vi "TestStand_Control ( Close_Seq ).vi"(8 "error in (no error)":errorcluster, 11 "TestStand UI Data":T1) -> (0 "error out":errorcluster)   [LabVIEW 2018, in "TestStand_Control.lvlib"]
uses:
  Module_Controls/TestStand UI Data.ctl
  TestStand_Control.lvlib
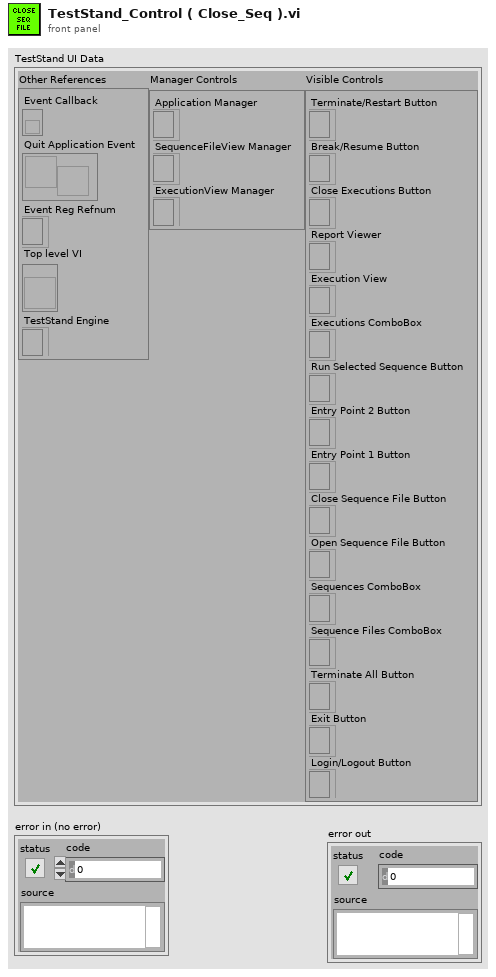
[diagram p1: front panel]
types:
  T1 = typedef "TestStand_Control.lvlib/TestStand UI Data.ctl" = cluster{"Other References":cluster{"Event Callback":refnum<k27>, "Quit Application Event":refnum<user-event>, "Event Reg Refnum":refnum<event-registration>, "Top level VI":refnum<vi>, "TestStand Engine":refnum<k7>}, "Manager Controls":cluster{"Application Manager":refnum<k7>, "SequenceFileView Manager":refnum<k7>, "ExecutionView Manager":refnum<k7>}, "Visible Controls":cluster{"Terminate/Restart Button":refnum<k7>, "Break/Resume Button":refnum<k7>, "Close Executions Button":refnum<k7>, "Report Viewer":refnum<k7>, "Execution View":refnum<k7>, "Executions ComboBox":refnum<k7>, "Run Selected Sequence Button":refnum<k7>, "Entry Point 2 Button":refnum<k7>, "Entry Point 1 Button":refnum<k7>, "Close Sequence File Button":refnum<k7>, "Open Sequence File Button":refnum<k7>, "Sequences ComboBox":refnum<k7>, "Sequence Files ComboBox":refnum<k7>, "Terminate All Button":refnum<k7>, "Exit Button":refnum<k7>, "Login/Logout Button":refnum<k7>}}
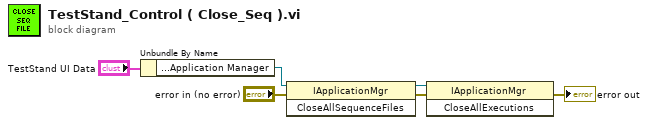
[diagram p0: block diagram]
diagram:
  n1 = Unbundle By Name("TestStand UI Data") -> ("Manager Controls.Application Manager"=w6:refnum<k7>)
  n2 = invoke class="IApplicationMgr" method="CloseAllSequenceFiles"(reference=w6, error in="error in (no error)") -> (reference out=w4:refnum<k7>, error out=w5:errorcluster)  [unwired: 1 in, 1 out]
  n3 = invoke class="IApplicationMgr" method="CloseAllExecutions"(reference=w4, error in=w5) -> (error out=→"error out":errorcluster)  [unwired: 1 in, 2 out]
